vi "Read LED Mode.vi"(8 "error in":errorcluster {"code" format="%.0x"}, 11 "Session In":refnum<visa-resource-name>) -> (0 "error out":errorcluster {"code" format="%.0x"}, 2 "Mode":i32, 3 "Session Out":refnum<visa-resource-name>)   [LabVIEW 2012, in "YOST 3 Space.lvlib"]
uses:
  YOST 3 Space.lvlib
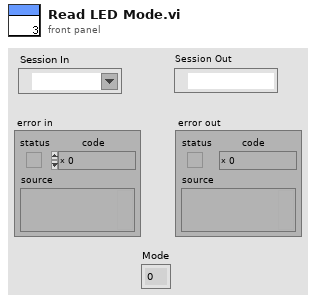
[diagram p1: front panel]
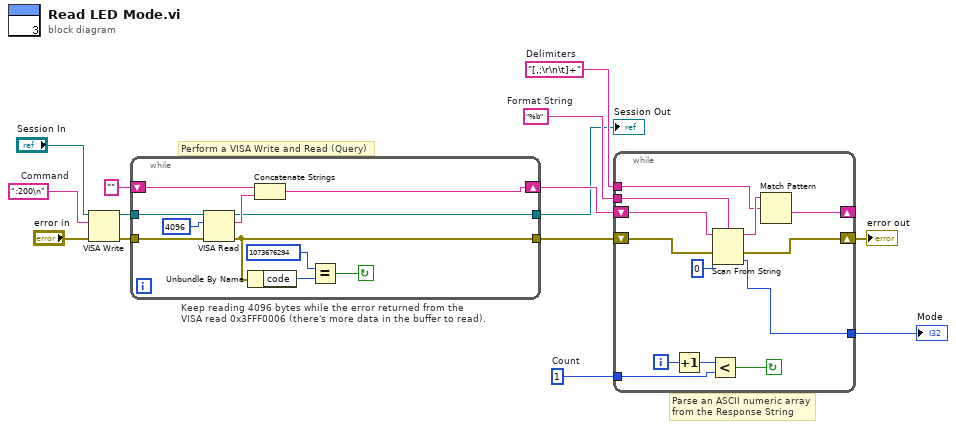
[diagram p0: block diagram]
diagram:
  w7 = "%b"  # Format String
  w6 = "[,;\r\n\t]+"  # Delimiters
  w8 = 1  # Count
  w10 = ":200\n"  # Command
  # "Parse an ASCII numeric array from the Response String"
  # "Perform a VISA Write and Read (Query)"
  # "Keep reading 4096 bytes while the error returned from the\nVISA read 0x3FFF0006 (there's more data in the buffer to read)."
  n1 = VISA Write(VISA resource name="Session In", write buffer=w10, error in (no error)="error in") -> (VISA resource name out=w14:refnum<visa-resource-name>, error out=w13:errorcluster)  [unwired: 1 out]
  n2 = while {
    tunnel: w14 -> [w22]
    shift-right: [w16] -> w9
    shift-left: "" -> [w21]
    tunnel: w13 -> [w19]
    tunnel: [w18] -> w12
    tunnel: [w15] -> w2
    stop <- w17 continue-if-true
    n3 = VISA Read(VISA resource name=w22, byte count=u32 4096 ("byte count (0)"), error in (no error)=w19) -> (VISA resource name out=w15:refnum<visa-resource-name>, read buffer=w20:string, error out=w18:errorcluster)  [unwired: 1 out]
    n4 = Unbundle By Name(w18) -> ("code"=w24:i32)
    n5 = Concatenate Strings(w21, w20) -> (w16:string)
    n6 = Equal?(x=1073676294, y=w24) -> (x = y?=w17:bool)
  }
  "Session Out" <- w2
  n7 = while {
    shift-right: [w30] -> _
    shift-left: w9 -> [w37]
    shift-right: [w29] -> w5
    shift-left: w12 -> [w36]
    tunnel: w8 -> [w33]
    tunnel: w7 -> [w32]
    tunnel: w6 -> [w28]
    tunnel: [w26] -> w1
    i -> [w35]
    stop <- w38 continue-if-true
    n8 = Increment(x=w35) -> (x+1=w34:i32)
    n9 = Less?(x=w34, y=w33) -> (x < y?=w38:bool)
    n10 = Scan From String(format string=w32, input string=w37, error in=w36, default 1=0 ("default value 2")) -> (remaining string=w31:string, error out=w29:errorcluster, output 1=w26:i32)  [unwired: 1 in, 1 out]
    n11 = Match Pattern(string=w31, regular expression=w28) -> (after substring=w30:string)  [unwired: 1 in, 3 out]
  }
  "error out" <- w5
  "Mode" <- w1
